vi "closeLog.vi"(8 "error in (no error)":errorcluster, 11 "Logger in":refnum<class "LoggerDatalog.lvclass">) -> (0 "error out":errorcluster, 3 "Logger out":refnum<class "LoggerDatalog.lvclass">)   [LabVIEW 2013, in "LoggerDatalog.lvclass"]
uses:
  LoggerDatalog.lvclass
  LoggerDatalog.lvclass/LoggerDatalog.ctl
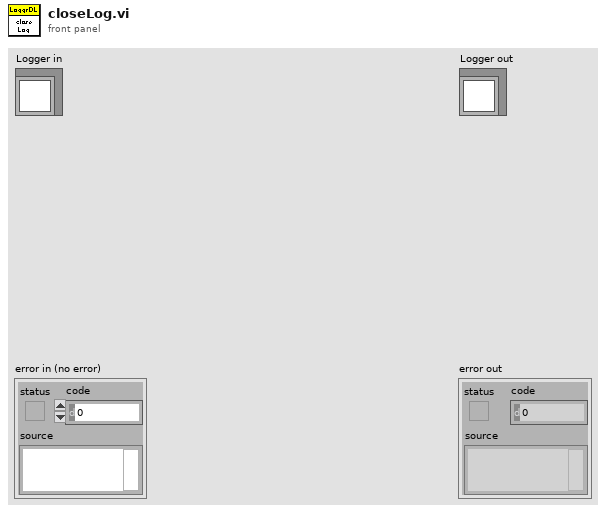
[diagram p1: front panel]
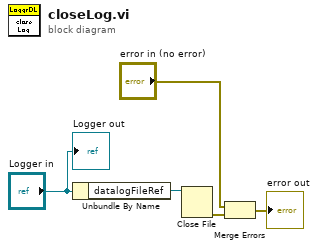
[diagram p0: block diagram]
diagram:
  n1 = Unbundle By Name("Logger in") -> ("datalogFileRef"=w4:refnum<k1>)
  n2 = Close File(refnum=w4) -> (error out=w2:errorcluster)  [unwired: 1 in, 1 out]
  n3 = Merge Errors("error in (no error)", w2) -> (→"error out":errorcluster)
  "Logger out" <- "Logger in"
